vi "LC1_main.vi"() -> ()   [LabVIEW 2016]
uses:
  LC1_Global.vi
  Communication/Global communication output.vi
  LabVIEW Data/MathScriptVIs/MCStatic_36913153632_2bc289e0a5f717e12810d9cf21ccd4a4.vi
  <instcachedir>/0/MCStatic_36913153632_2bc289e0a5f717e12810d9cf21ccd4a4_D477B428622C441095E26A127D1E036B.lvgen/MCStatic_36913153632_2bc289e0a5f717e12810d9cf21ccd4a4_D477B428622C441095E26A127D1E036B_000.vi
  <vilib>/imath/engines/lvmath2/RunTimeEngine/BuiltInFunctions/abs/NIMS_abs(unsigned).vi
  <instcachedir>/0/NIMS_abs(unsigned)_CB0E2CC90712458C87FBF103B22FBEA1.lvgen/NIMS_abs(unsigned)_CB0E2CC90712458C87FBF103B22FBEA1_002.vi
  <vilib>/imath/engines/lvmath2/RunTimeEngine/NodeEndStatement/NIMS_NodeEndStatement_Output.vi
  <instcachedir>/0/NIMS_NodeEndStatement_Output_53EC0D466D134D7ABD903AC30B43404B.lvgen/NIMS_NodeEndStatement_Output_53EC0D466D134D7ABD903AC30B43404B_001.vi
  <vilib>/imath/engines/lvmath2/RunTimeEngine/ErrorHandling/NIMS_Finalize Error.vi
  <vilib>/ErrorRing/Error Ring.xnode
  BESS_LC/PIcontroller.m
panel:
  in  "y":dbl=0.05
  in  "p_in":dbl=0.2
  in  "i_in":dbl=0.2
  in  "p_an":dbl
  in  "i_an":dbl=0.01
  out "error out":errorcluster
  in  "Enable":bool=TRUE
  in  "i_mag":dbl=0.1
  in  "p_mag":dbl=0.1
  out "MGCC_to_BESS":dbl[](array[numeric])=[1.0, 0.0, 0.0, 1.998884210188606, -0.007911213321293431, 6.679101716144942e-12, 1.8051253380946264e-08, -2.7375026689924198e-09, 0.0, 0.0] format="%#_6f"
  out "Waveform Chart 2":dbl(graph)=-1.8051253380946264e-08
  out "Waveform Chart":dbl[][](graph)=[[-2.7375026689924198e-09, 1.9988842101912097, -6.679101716144942e-12]]
  in  "LC1_WatchDogTimer Enable":bool=TRUE
  # "Copyright <2020> <The University of Tennessee at Knoxville and the University of Tennessee Research Foundation>\n\nRedistribution and use in source and binary forms, with or without modification, are permitted provided that the following conditions are met:\n\n1. Redistributions of source code must retain the above copyright notice, this list of conditions and the following disclaimer.\n\n2. Redistributions in binary form must reproduce the above copyright notice, this list of conditions and the following disclaimer in the documentation and/or other materials provided with the distribution.\n\n3. Neither the name of the copyright holder nor the names of its contributors may be used to endorse or promote products derived from this software without specific prior written permission.\n\nTHIS SOFTWARE IS PROVIDED BY THE COPYRIGHT HOLDERS AND CONTRIBUTORS \"AS IS\" AND ANY EXPRESS OR IMPLIED WARRANTIES, INCLUDING, BUT NOT LIMITED TO, THE IMPLIED WARRANTIES OF MERCHANTABILITY AND FITNESS FOR A PARTICULAR PURPOSE ARE DISCLAIMED. IN NO EVENT SHALL THE COPYRIGHT HOLDER OR CONTRIBUTORS BE LIABLE FOR ANY DIRECT, INDIRECT, INCIDENTAL, SPECIAL, EXEMPLARY, OR CONSEQUENTIAL DAMAGES (INCLUDING, BUT NOT LIMITED TO, PROCUREMENT OF SUBSTITUTE GOODS OR SERVICES; LOSS OF USE, DATA, OR PROFITS; OR BUSINESS INTERRUPTION) HOWEVER CAUSED AND ON ANY THEORY OF LIABILITY, WHETHER IN CONTRACT, STRICT LIABILITY, OR TORT (INCLUDING NEGLIGENCE OR OTHERWISE) ARISING IN ANY WAY OUT OF THE USE OF THIS SOFTWARE, EVEN IF ADVISED OF THE POSSIBILITY OF SUCH DAMAGE."
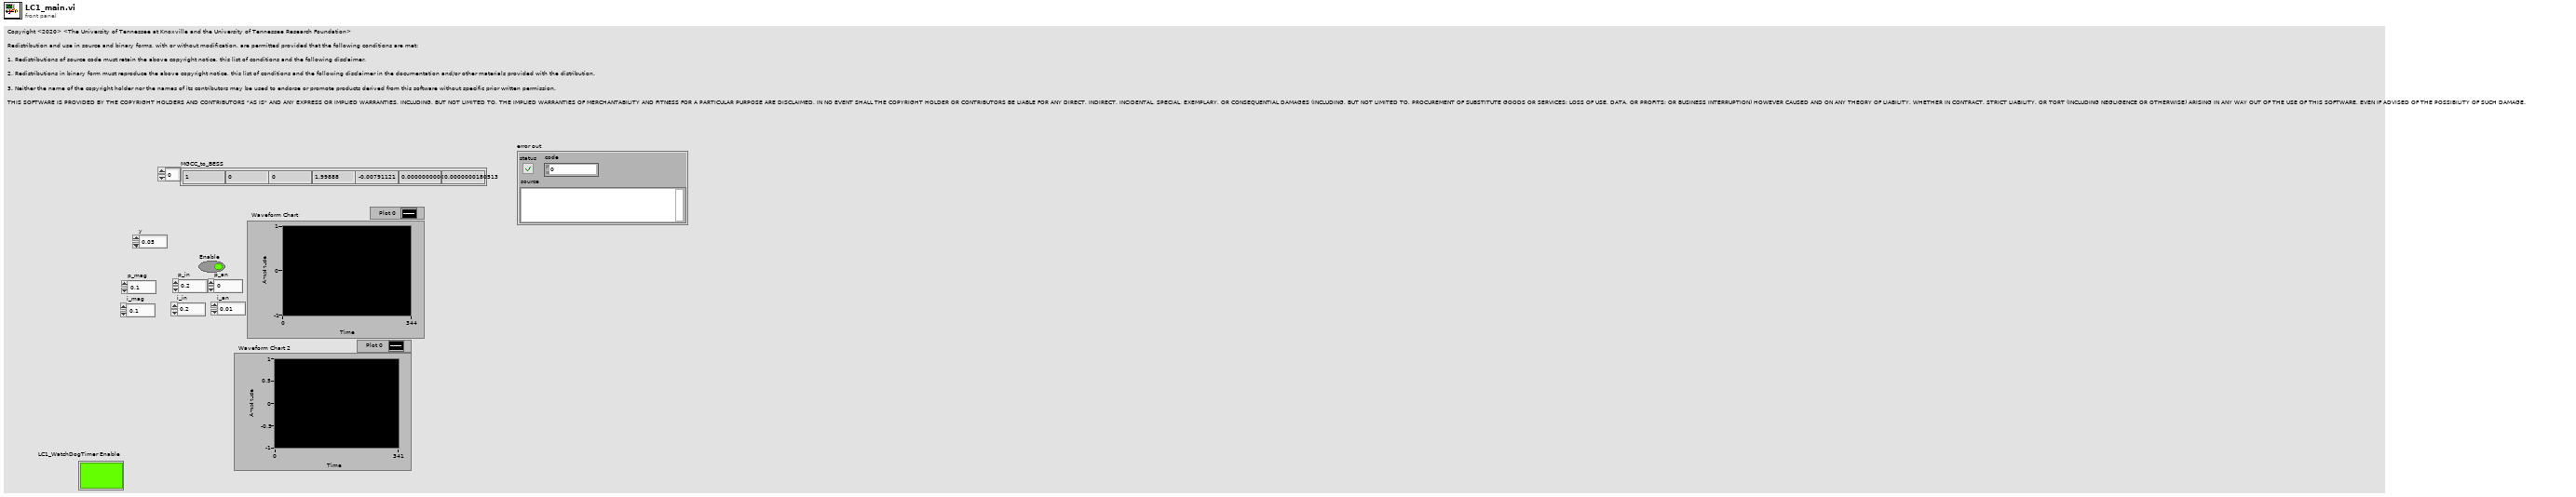
[diagram p1: front panel]
types:
  T1 = typedef "NI_Matrix.lvlib/RealMatrix.ctl" = dbl[][]
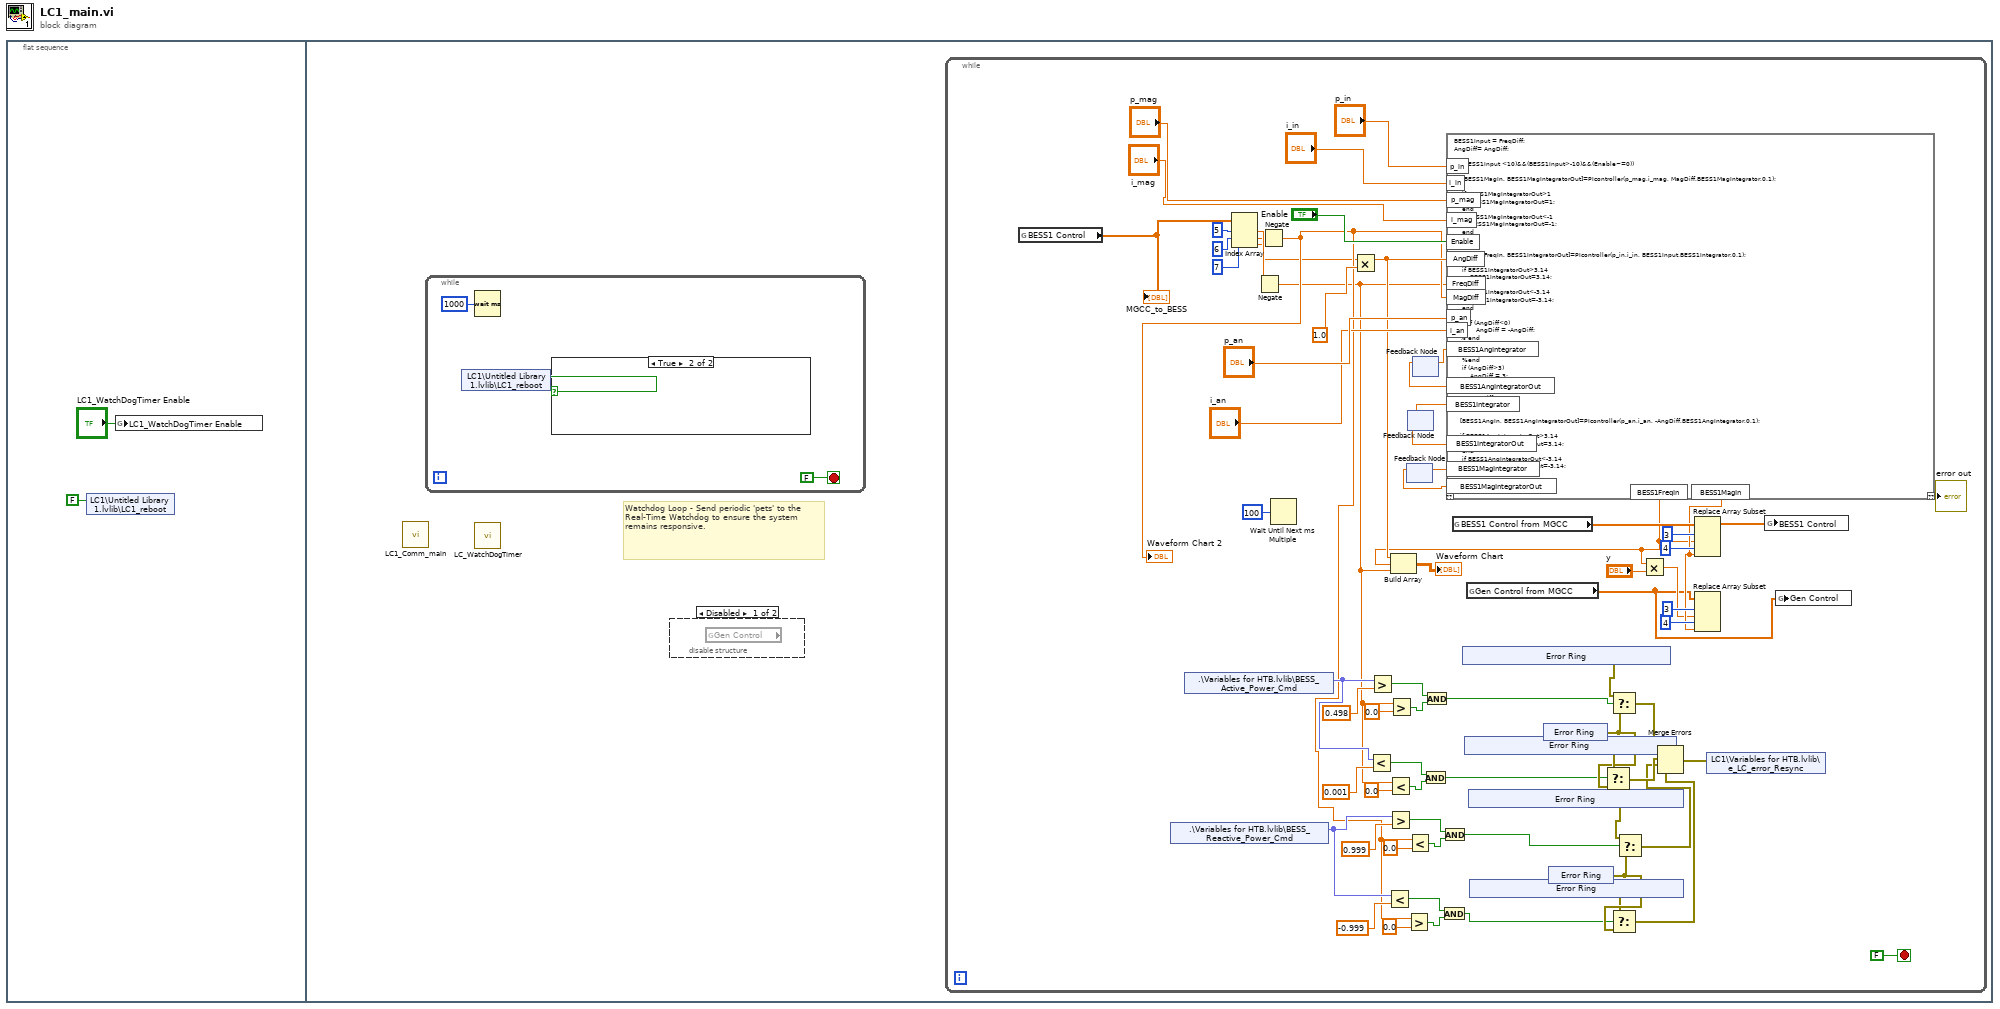
[diagram p0: block diagram]
diagram:
  n1 = flat-sequence {
    frame #0 {
      n2 = shared-variable "LC1\\Untitled Library 1.lvlib\\LC1_reboot"(FALSE ("LC1_reboot")) -> ()  [unwired: 1 in, 1 out]
      n3 = global write "LC1_Global.vi" "LC1_WatchDogTimer Enable"("LC1_WatchDogTimer Enable") -> ()
    }
    frame #1 {
      # "Watchdog Loop - Send periodic 'pets' to the Real-Time Watchdog to ensure the system remains responsive."
      n4 = call "LC1_Comm_main.vi"() -> ()  [unwired: 12 in]
      n5 = while {
        stop <- FALSE stop-if-true
        n6 = shared-variable "LC1\\Untitled Library 1.lvlib\\LC1_reboot"() -> (w534:bool)  [unwired: 1 in, 1 out]
        n7 = Wait (ms)(milliseconds to wait=u32 1000) -> ()  [unwired: 1 out]
        n8 = case shown="True" w534 {
          frame False {
          }
          frame True {
          }
        }
      }
      n9 = call "LC_WatchDogTimer.vi"() -> ()  [unwired: 12 in]
      n10 = disable-structure shown="Disabled" {
        frame Disabled {
          n11 = global read "Global communication output.vi" "Gen Control"() -> ()  [unwired: 1 out]
        }
        frame Enabled {
        }
      }
      n12 = while {
        stop <- FALSE stop-if-true
        n13 = global read "Global communication output.vi" "BESS1 Control"() -> (w19:dbl[])
        "MGCC_to_BESS" <- w19
        n14 = shared-variable ".\\Variables for HTB.lvlib\\BESS_Reactive_Power_Cmd"() -> (w27:fxp<+/-,64,32>)  [unwired: 1 in, 1 out]
        n15 = shared-variable ".\\Variables for HTB.lvlib\\BESS_Active_Power_Cmd"() -> (w28:fxp<+/-,64,32>)  [unwired: 1 in, 1 out]
        n16 = Index Array(array=w19, index #1=5 ("index"), index #2=6 ("index"), index #3=7 ("index")) -> (element #1=w14:dbl, element #2=w13:dbl, element #3=w10:dbl)
        n17 = Negate(x=w14) -> (-x=w11:dbl)
        n18 = Negate(x=w13) -> (-x=w12:dbl)
        "Waveform Chart 2" <- w12
        n19 = Wait Until Next ms Multiple(millisecond multiple=u32 100) -> ()  [unwired: 1 out]
        n20 = Multiply(x=w10, y=1.0) -> (x*y=w53:dbl)
        n21 = Less?(x=w28, y=0.001 ("upper limit")) -> (x < y?=w39:bool)
        n22 = Greater?(x=w28, y=0.498 ("upper limit")) -> (0:w51:bool)
        n23 = Less?(x=w27, y=-0.999 ("upper limit")) -> (x < y?=w35:bool)
        n24 = Less?(x=w11, y=0.0) -> (x < y?=w41:bool)
        n25 = Greater?(x=w27, y=0.999 ("upper limit")) -> (0:w30:bool)
        n26 = Greater?(x=w11, y=0.0) -> (0:w49:bool)
        n27 = feedback #1() -> (w55:dbl)  [unwired: 1 in]
        n28 = Greater?(x=w12, y=0.0) -> (0:w33:bool)
        n29 = Less?(x=w12, y=0.0) -> (x < y?=w32:bool)
        n30 = feedback #2() -> (w73:dbl)  [unwired: 1 in]
        n31 = feedback #3() -> (w70:dbl)  [unwired: 1 in]
        n32 = And(x=w39, y=w41) -> (x .and. y?=w37:bool)
        n33 = And(x=w51, y=w49) -> (x .and. y?=w42:bool)
        n34 = And(x=w35, y=w33) -> (x .and. y?=w20:bool)
        n35 = And(x=w30, y=w32) -> (x .and. y?=w21:bool)
        n36 = mathscript code="BESS1Input = FreqDiff;\nAngDiff= AngDiff;\n\nif ((BESS1Input <10)&&(BESS1Input>-10)&&(Enable~=0))\n\n    [BESS1MagIn, BESS1MagIntegratorOut]=PIcontroller(p_mag,i_mag, MagDiff,BESS1MagIntegrator,0.1);\n   \n    if BESS1MagIntegratorOut>1\n        BESS1MagIntegratorOut=1;\n    end\n    if BESS1MagIntegratorOut<-1\n        BESS1MagIntegratorOut=-1;\n    end\n\n\n    [BESS1FreqIn, BESS1IntegratorOut]=PIcontroller(p_in,i_in, BESS1Input,BESS1Integrator,0.1);\n   \n    if BESS1IntegratorOut>3.14\n        BESS1IntegratorOut=3.14;\n    end\n    if BESS1IntegratorOut<-3.14\n        BESS1IntegratorOut=-3.14;\n    end\n\n%    if (AngDiff<0)\n %       AngDiff = -AngDiff;\n   % end \n    %if (AngDiff> 5)\n     %   AngDiff = 0;\n    %end \n    if (AngDiff>3)\n        AngDiff = 3;\n    end \n    if (AngDiff<-3)\n        AngDiff = -3;\n    end \n\n   [BESS1AngIn, BESS1AngIntegratorOut]=PIcontroller(p_an,i_an, -AngDiff,BESS1AngIntegrator,0.1);\n\n   if BESS1AngIntegratorOut>3.14\n        BESS1AngIntegratorOut=3.14;\n    end\n    if BESS1AngIntegratorOut<-3.14\n        BESS1AngIntegratorOut=-3.14;\n    end\n    \n    if abs(FreqDiff<0.2)\n        BESS1FreqIn = BESS1FreqIn + BESS1AngIn;\n    else\n        BESS1AngIntegratorOut = 0;\n    end\n    if (BESS1FreqIn > 3.14) \n          BESS1FreqIn = 3.14;\n    end\n    if (BESS1FreqIn < -3.14) \n          BESS1FreqIn = -3.14;\n    end\n\n    if (AngDiff ==0)&&(FreqDiff == 0) && (MagDiff== 0)\n        BESS1FreqIn = 0;\n        BESS1MagIn = 0;\n        BESS1IntegratorOut = 0;\n        BESS1MagIntegratorOut = 0;\n        BESS1AngIntegratorOut = 0;\n    end\n\nelse\nBESS1FreqIn = 0;\nBESS1MagIn = 0;\nBESS1IntegratorOut = 0;\nBESS1MagIntegratorOut = 0;\nBESS1AngIntegratorOut = 0;\nend"("AngDiff"=w53, "BESS1Integrator"=w73, "FreqDiff"=w11, "BESS1AngIntegrator"=w70, "Enable"="Enable", "p_in"="p_in", "i_in"="i_in", "p_an"="p_an", "i_an"="i_an", "p_mag"="p_mag", "i_mag"="i_mag", "BESS1MagIntegrator"=w55, "MagDiff"=w12) -> ("??"=→"error out":errorcluster, "BESS1IntegratorOut"=w72:dbl, "BESS1FreqIn"=w5:dbl, "BESS1AngIntegratorOut"=w71:dbl, "BESS1MagIntegratorOut"=w56:dbl, "BESS1MagIn"=w7:dbl)  [unwired: 1 in]
        n37 = Build Array(w53, w5, w11) -> (→"Waveform Chart":T1)
        n38 = feedback-in #1(w56) -> ()
        n39 = feedback-in #2(w72) -> ()
        n40 = feedback-in #3(w71) -> ()
        n41 = global read "Global communication output.vi" "BESS1 Control from MGCC"() -> (w18:dbl[])
        n42 = xnode "Error Ring"() -> ("error out"=w47:errorcluster)
        n43 = xnode "Error Ring"() -> ("error out"=w45:errorcluster)
        n44 = global read "Global communication output.vi" "Gen Control from MGCC"() -> (w3:dbl[])
        n45 = xnode "Error Ring"() -> ("error out"=w24:errorcluster)
        n46 = xnode "Error Ring"() -> ("error out"=w25:errorcluster)
        n47 = xnode "Error Ring"() -> ("error out"=w43:errorcluster)
        n48 = xnode "Error Ring"() -> ("error out"=w26:errorcluster)
        n49 = Select(t=w45, s=w37, f=w43) -> (s? t:f=w44:errorcluster)
        n50 = Select(t=w47, s=w42, f=w43) -> (s? t:f=w46:errorcluster)
        n51 = Select(t=w25, s=w20, f=w26) -> (s? t:f=w22:errorcluster)
        n52 = Select(t=w24, s=w21, f=w26) -> (s? t:f=w23:errorcluster)
        n53 = Multiply(x=w5, y="y") -> (x*y=w6:dbl)
        n54 = Merge Errors(w46, w44, w23, w22) -> (w48:errorcluster)
        n55 = Replace Array Subset(array=w18, new element #1=w5, index #1=3 ("index"), new element #2=w7, index #2=4 ("index")) -> (w15:dbl[])
        n56 = Replace Array Subset(array=w3, new element #1=w6, index #1=3 ("index"), new element #2=w7, index #2=4 ("index")) -> ()  [unwired: 1 out]
        n57 = shared-variable "LC1\\Variables for HTB.lvlib\\e_LC_error_Resync"(w48) -> ()  [unwired: 1 in, 1 out]
        n58 = global write "Global communication output.vi" "BESS1 Control"(w15) -> ()
        n59 = global write "Global communication output.vi" "Gen Control"(w3) -> ()
      }
    }
  }
